vi "Tukey.vi"(4 "f2 (MHz)":dbl=80.0 format="%0.2f", 5 "Pk Value":i32=1, 6 "f1 (MHz)":dbl=10.0 format="%0.2f", 7 "Samp Rate (mics)":dbl=1.0 min=1.0 max=1190.0, 8 "Pts":u16, 10 "Tukey":dbl=0.15, 11 "Lobe ratio":dbl=90.0) -> (2 "Tukey Chirp":dbl[](graph), 3 "Tukey Window":dbl[](graph))   [LabVIEW 2022 SP3]
uses:
  <vilib>/Analysis/4window.llb/Chebyshev Window (DBL).vi
  <vilib>/Analysis/NI_AALPro.lvlib
  <vilib>/Analysis/NI_AALBase.lvlib
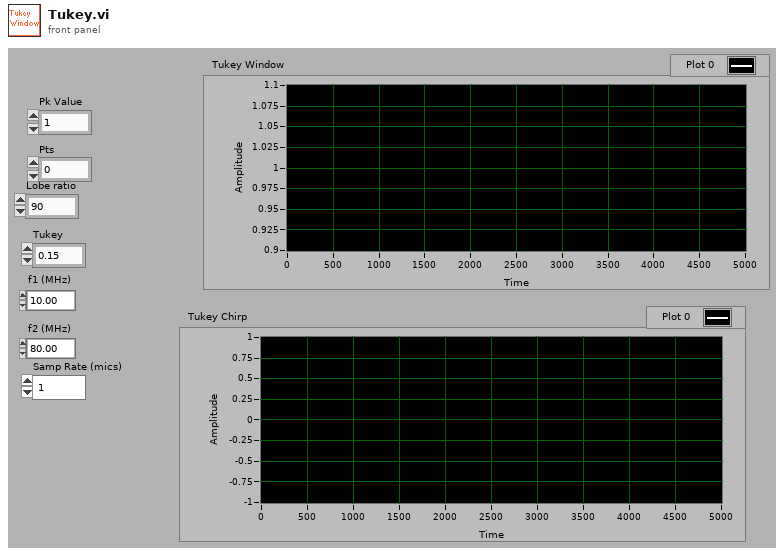
[diagram p1: front panel]
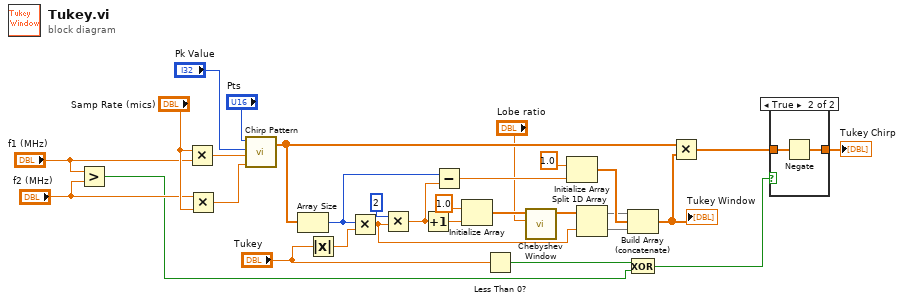
[diagram p0: block diagram]
diagram:
  n1 = Greater?(x="f1 (MHz)", y="f2 (MHz)") -> (0:w5:bool)
  n2 = Multiply(x="Samp Rate (mics)", y="f1 (MHz)") -> (x*y=w27:dbl)
  n3 = Multiply(x="f2 (MHz)", y="Samp Rate (mics)") -> (x*y=w28:dbl)
  n4 = call <vilib>:"Chirp Pattern.vi"("f2"=w28, "f1"=w27, "amplitude"="Pk Value", "samples"="Pts") -> ("Chirp Pattern"=w9:dbl[])  [unwired: 1 out]
  n5 = Array Size(array=w9) -> (size(s)=w21:i32)
  n6 = Absolute Value(x="Tukey") -> (abs(x)=w2:dbl)
  n7 = Multiply(x=w21, y=w2) -> (x*y=w19:dbl)
  n8 = Multiply(x=2, y=w19) -> (x*y=w18:dbl)
  n9 = Increment(x=w18) -> (x+1=w13:dbl)
  n10 = Subtract(x=w21, y=w18) -> (x-y=w23:dbl)
  n11 = Initialize Array(1.0 ("element"), w13) -> (w25:dbl[])
  n12 = Less Than 0?(x="Tukey") -> (x < 0?=w6:bool)
  n13 = call-poly <vilib>:"Chebyshev Window.vi"("lobe ratio (dB)"="Lobe ratio", "X"=w25) -> ("Windowed X"=w22:dbl[])  [unwired: 9 out]
  n14 = Initialize Array(1.0 ("element"), w23) -> (w17:dbl[])
  n15 = Split 1D Array(array=w22, index=w19) -> (first subarray=w16:dbl[], second subarray=w15:dbl[])
  n16 = Build Array (concatenate)(w16, w17, w15) -> (w14:dbl[])
  "Tukey Window" <- w14
  n17 = Exclusive Or(1:w5, 2:w6) -> (0:w4:bool)
  n18 = Multiply(x=w9, y=w14) -> (x*y=w8:dbl[])
  n19 = case shown="True" w4 {
    tunnel: [w31 w32] -> w7
    tunnel: w8 -> [w31 w33]
    frame False {
    }
    frame True {
      n20 = Negate(x=w33) -> (-x=w32:dbl[])
    }
  }
  "Tukey Chirp" <- w7
